vi "NC Motor GS LV.vi"() -> ()   [LabVIEW 2014]
uses:
  F:/Labview GS ver 2014/NCmotorGSLV.dll
  NCmotorGSLV.dll
  <vilib>/Instr/_visa.llb/VISA Configure Serial Port (Instr).vi
panel:
  out "SoftVer":string caption="Controller Software ver"
  in  "Baud Rate":T1(radio)=enum."9600"
  in  "StopAll":bool caption="Stop Motor"
  out "VerInfo":string caption="DLL Version"
  in  "stop":bool
  in  "VISA resource name":refnum<visa-resource-name> caption="Select Serial Port"
  in  "Serial Port":bool
  in  "M1Init":bool
  in  "M1Home":bool
  in  "M1HomeTo":T2(radio) caption="Home To"
  in  "b1SP1":bool
  in  "b1SP9":bool
  in  "b1SP8":bool
  in  "b1SP7":bool
  in  "b1SP6":bool
  in  "b1SP5":bool
  in  "b1SP4":bool
  in  "b1SP3":bool
  in  "b1SP2":bool
  in  "b1SP0":bool
  out "M1SP9":string caption="SP1"
  out "M1SP8":string caption="SP1"
  out "M1SP7":string caption="SP1"
  out "M1SP6":string caption="SP1"
  out "M1SP5":string caption="SP1"
  out "M1SP4":string caption="SP1"
  out "M1SP3":string caption="SP1"
  out "M1SP2":string caption="SP1"
  out "M1SP1":string caption="SP1"
  out "M1SP0":string caption="SP0"
  in  "StopM1":bool caption="Stop Motor"
  out "MovingM1":bool caption="Moving"
  out "ErrorM1":bool caption="Pos Error"
  out "InitM1":bool caption="Not Initialised"
  out "HomeM1":bool caption="Not Homed"
  out "ReadyM1":bool caption="Ready"
  in  "NewAccelM1":u16 caption="New Acceleration" max=5000
  in  "NewVelM1":u16 caption="New Velocity" max=5000
  out "AccelM1":string caption="Acceleration"
  out "VelM1":string caption="Velocity"
  in  "M1Send":bool
  in  "AddM1":u8=1 caption="Address" min=1 max=15 step=1 format="%x"
  out "PosM1":string caption="Position"
  in  "NewPosM1":i32 caption="New Position"
  in  "Motor1On":bool caption="Enable"
  in  "M2Init":bool
  in  "M2Home":bool
  in  "M2HomeTo":T2(radio) caption="Home To"
  out "M2SP8":string caption="SP1"
  out "M2SP9":string caption="SP1"
  out "M2SP7":string caption="SP1"
  out "M2SP6":string caption="SP1"
  out "M2SP5":string caption="SP1"
  out "M2SP4":string caption="SP1"
  out "M2SP3":string caption="SP1"
  in  "b2SP2":bool
  in  "b2SP9":bool
  in  "b2SP8":bool
  in  "b2SP7":bool
  in  "b2SP6":bool
  in  "b2SP5":bool
  in  "b2SP4":bool
  out "M2SP2":string caption="SP1"
  in  "b2SP3":bool
  in  "b2SP1":bool
  in  "b2SP0":bool
  out "M2SP1":string caption="SP1"
  out "M2SP0":string caption="SP0"
  in  "StopM2":bool caption="Stop Motor"
  in  "NewAccelM2":u16 caption="New Acceleration" max=5000
  in  "NewVelM2":u16 caption="New Velocity" max=5000
  out "AccelM2":string caption="Acceleration"
  out "VelM2":string caption="Velocity"
  in  "M2Send":bool caption="M1Send"
  out "PosM2":string caption="Position"
  in  "NewPosM2":i32 caption="New Position"
  out "MovinM2":bool caption="Moving"
  out "ErrorM2":bool caption="Pos Error"
  out "InitM2":bool caption="Not Initialised"
  out "HomeM2":bool caption="Not Home"
  out "ReadyM2":bool caption="Ready"
  in  "AddM2":u8=2 caption="Address" min=1 max=15
  in  "Motor2On":bool caption="Enable"
  in  "M3Init":bool
  in  "M3Home":bool
  in  "M3HomeTo":T2(radio) caption="Home To"
  out "M3SP9":string caption="SP1"
  out "M3SP8":string caption="SP1"
  out "M3SP7":string caption="SP1"
  out "M3SP6":string caption="SP1"
  out "M3SP5":string caption="SP1"
  out "M3SP4":string caption="SP1"
  out "M3SP3":string caption="SP1"
  in  "b3SP2":bool
  in  "b3SP9":bool
  in  "b3SP8":bool
  in  "b3SP7":bool
  in  "b3SP6":bool
  in  "b3SP5":bool
  in  "b3SP4":bool
  out "M3SP2":string caption="SP1"
  in  "b3SP3":bool
  in  "b3SP1":bool
  in  "b3SP0":bool
  out "M3SP1":string caption="SP1"
  out "M3SP0":string caption="SP0"
  in  "StopM3":bool caption="Stop Motor"
  in  "NewAccelM3":u16 caption="New Acceleration" max=5000
  in  "NewVelM3":u16 caption="New Velocity" max=5000
  out "AccelM3":string caption="Acceleration"
  out "VelM3":string caption="Velocity"
  in  "M3Send":bool caption="M1Send"
  out "PosM3":string caption="Position"
  in  "NewPosM3":i32 caption="New Position"
  out "MovinM3":bool caption="Moving"
  out "ErrorM3":bool caption="Pos Error"
  out "InitM3":bool caption="Not Initialised"
  out "HomeM3":bool caption="Not Home"
  out "ReadyM3":bool caption="Ready"
  in  "AddM3":u8=3 caption="Address" min=1 max=15
  in  "Motor3On":bool caption="Enable"
  out "error out":errorcluster
  out "RxData":string
  # "NC Motor GS LV.vi"
  # "2.  Select Baud rate"
  # "3.  Set motor address"
  # "4.  Enable motors"
  # "1.  Select COM port"
  # "5.  Open serial port"
  # "Set Points"
  # "Motor 1"
  # "Set Points"
  # "Motor 2"
  # "Set Points"
  # "Motor 3"
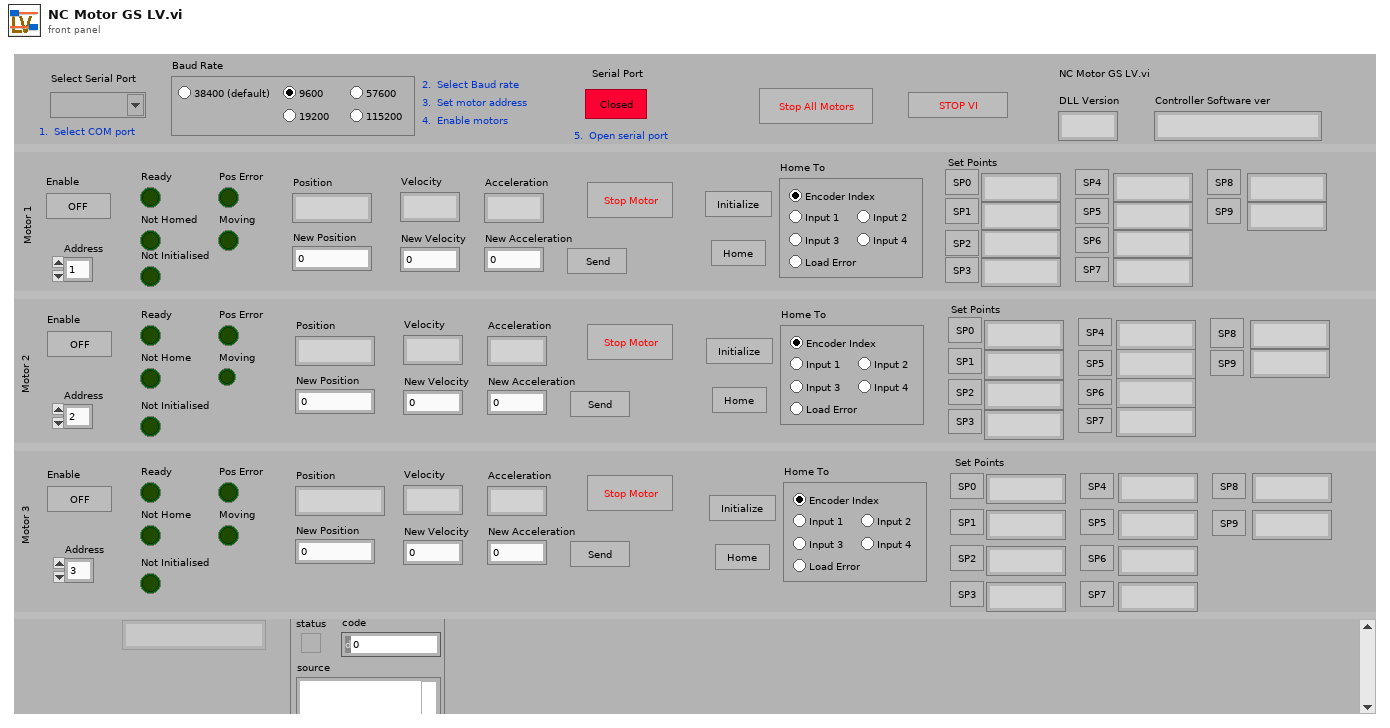
[diagram p1: front panel]
types:
  T1 = enum32{"No Selection", "9600", "19200", "38400", "57600", "115200"}
  T2 = enum32{"Enc", "Input1", "Input2", "Input3", "Input4", "Load"}
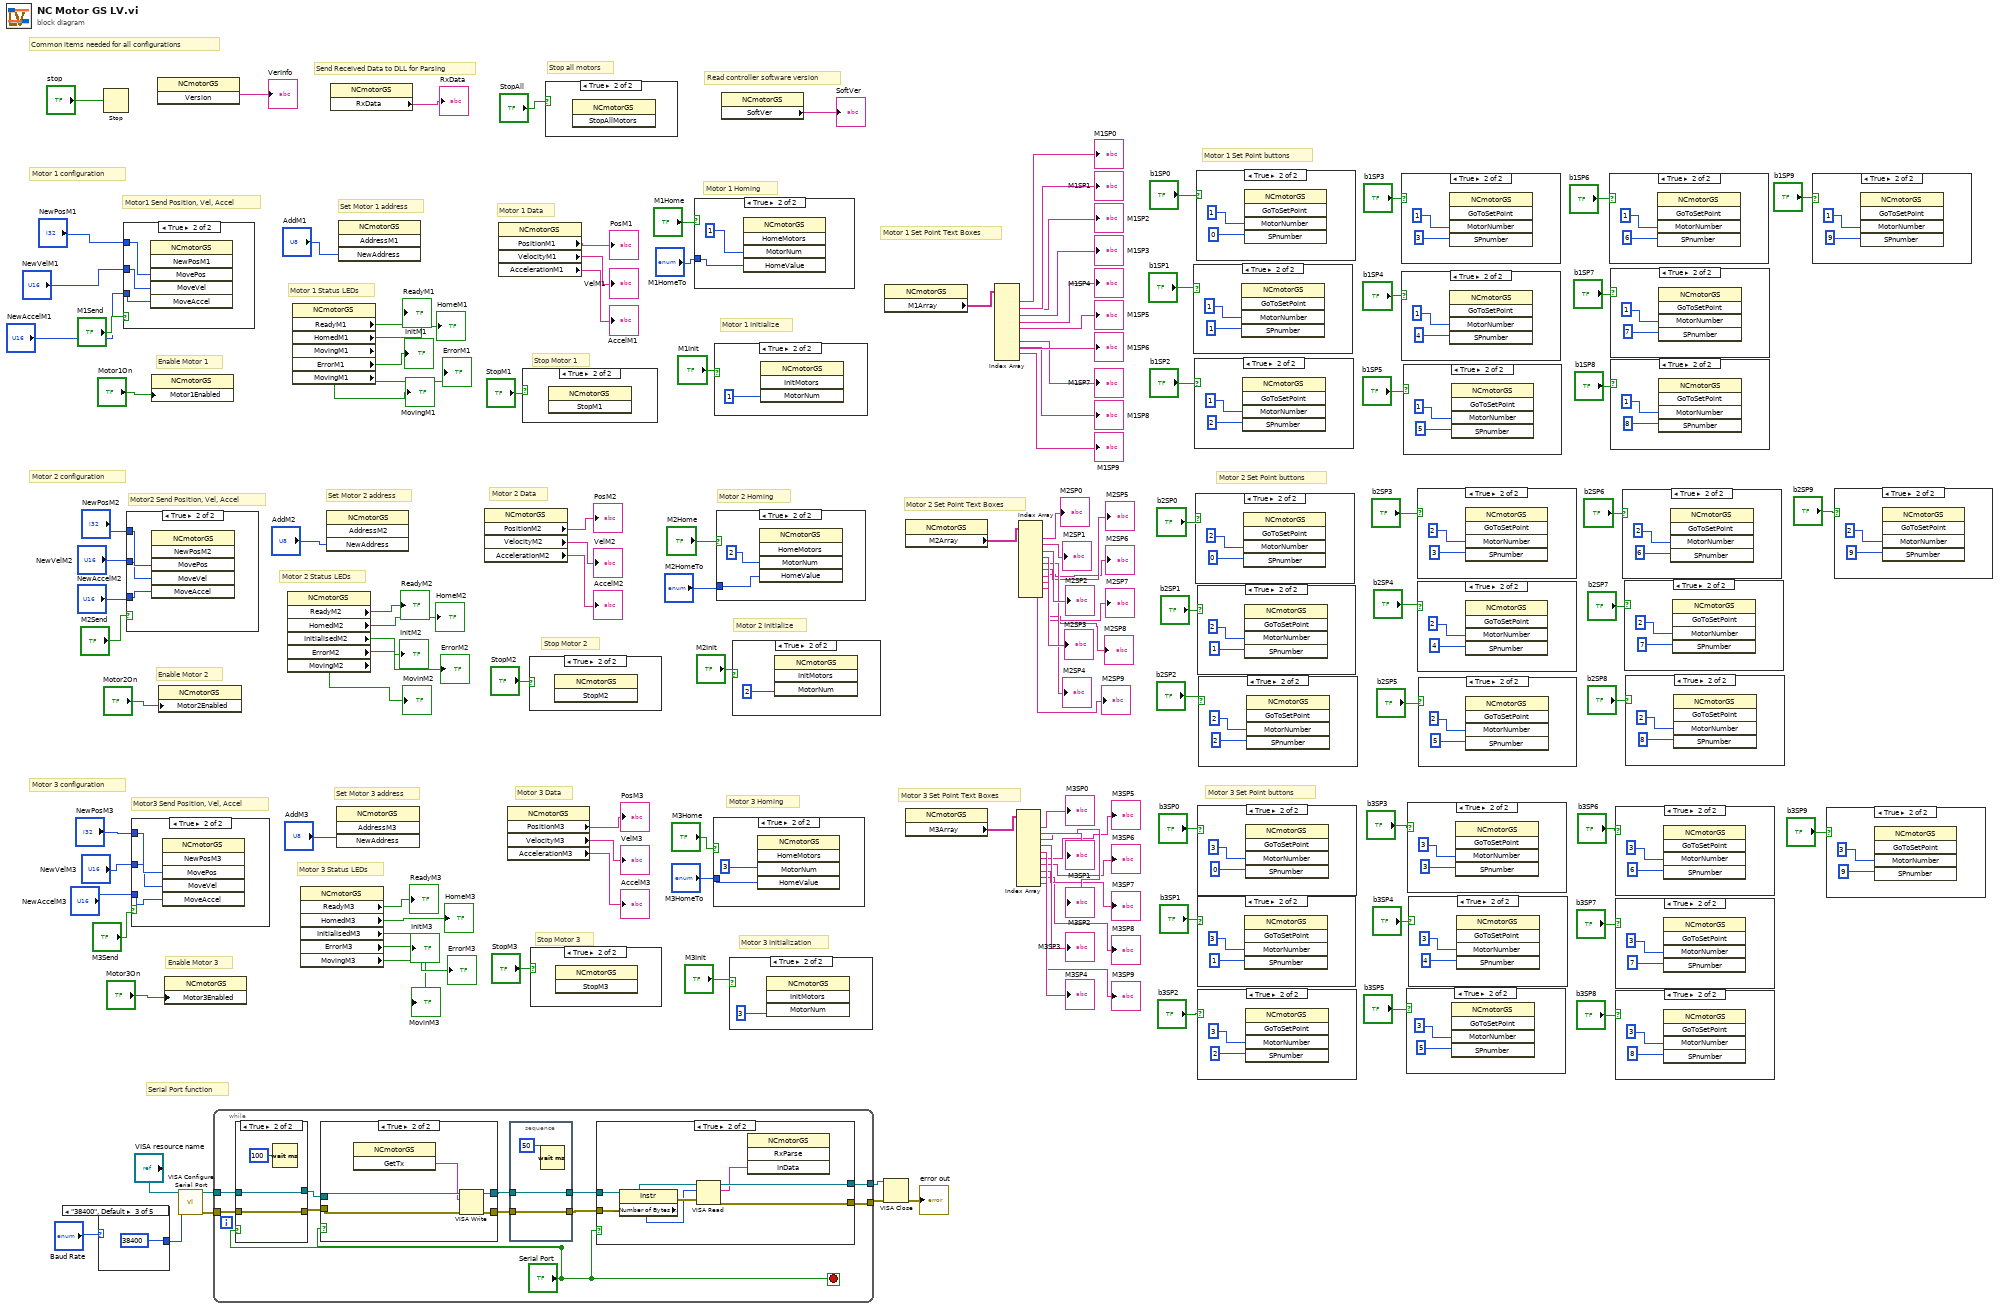
[diagram p0: block diagram]
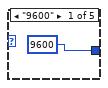
[diagram p11: hidden frame]
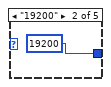
[diagram p12: hidden frame]
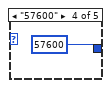
[diagram p13: hidden frame]
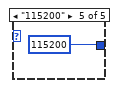
[diagram p14: hidden frame]
diagram:
  # "Read controller software version"
  # "Serial Port function"
  # "Motor 3 Homing"
  # "Motor 3 Initialization"
  # "Motor 2 Homing"
  # "Motor 2 Initialize"
  # "Motor 1 Initialize"
  # "Motor 1 Homing"
  # "Motor 3 Set Point buttons"
  # "Motor 2 Set Point buttons"
  # "Motor 1 Set Point buttons"
  # "Enable Motor 3"
  # "Enable Motor 2"
  # "Enable Motor 1"
  # "Stop Motor 1"
  # "Stop Motor 2"
  # "Stop Motor 3"
  # "Set Motor 3 address"
  # "Set Motor 2 address"
  # "Set Motor 1 address"
  # "Motor 3 configuration"
  # "Motor 1 Data"
  # "Motor 2 configuration"
  # "Motor 1 configuration"
  # "Common items needed for all configurations"
  # "Motor3 Send Position, Vel, Accel"
  # "Motor2 Send Position, Vel, Accel"
  # "Send Received Data to DLL for Parsing"
  # "Motor 2 Data"
  # "Motor 3 Data"
  # "Motor 1 Status LEDs"
  # "Motor 2 Status LEDs"
  # "Motor 3 Status LEDs"
  # "Motor 3 Set Point Text Boxes"
  # "Motor 2 Set Point Text Boxes"
  # "Motor1 Send Position, Vel, Accel"
  # "Stop all motors"
  # "Motor 1 Set Point Text Boxes"
  n1 = case shown="\"38400\", Default" "Baud Rate" {
    tunnel: [u32 9600 u32 19200 u32 38400 u32 57600 u32 115200] -> w18
    frame "9600" {
    }
    frame "19200" {
    }
    frame "38400", Default {
    }
    frame "57600" {
    }
    frame "115200" {
    }
  }
  n2 = Stop(stop? (T)="stop") -> ()
  n3 = case shown="True" "M1Send" {
    tunnel: "NewPosM1" -> [_ w138]
    tunnel: "NewVelM1" -> [_ w137]
    tunnel: "NewAccelM1" -> [_ w136]
    frame False {
    }
    frame True {
      n4 = invoke class="NCmotorGS" method="NewPosM1"("MovePos"=w138, "MoveVel"=w137, "MoveAccel"=w136) -> ()  [unwired: 3 in, 6 out]
    }
  }
  n5 = case shown="True" "M2Send" {
    tunnel: "NewPosM2" -> [_ w141]
    tunnel: "NewVelM2" -> [_ w140]
    tunnel: "NewAccelM2" -> [_ w139]
    frame False {
    }
    frame True {
      n6 = invoke class="NCmotorGS" method="NewPosM2"("MovePos"=w141, "MoveVel"=w140, "MoveAccel"=w139) -> ()  [unwired: 3 in, 6 out]
    }
  }
  n7 = case shown="True" "M3Send" {
    tunnel: "NewPosM3" -> [_ w144]
    tunnel: "NewVelM3" -> [_ w143]
    tunnel: "NewAccelM3" -> [_ w142]
    frame False {
    }
    frame True {
      n8 = invoke class="NCmotorGS" method="NewPosM3"("MovePos"=w144, "MoveVel"=w143, "MoveAccel"=w142) -> ()  [unwired: 3 in, 6 out]
    }
  }
  n9 = property class="NCmotorGS"("Motor1Enabled"="Motor1On") -> ()  [unwired: 2 in, 2 out]
  n10 = invoke class="NCmotorGS" method="Version"() -> ("Version"=→"VerInfo":string)  [unwired: 3 in, 2 out]
  n11 = property class="NCmotorGS"("Motor2Enabled"="Motor2On") -> ()  [unwired: 2 in, 2 out]
  n12 = property class="NCmotorGS"("Motor3Enabled"="Motor3On") -> ()  [unwired: 2 in, 2 out]
  n13 = call-poly "VISA Configure Serial Port"("VISA resource name"="VISA resource name", "baud rate (9600)"=w18) -> ("VISA resource name out"=w7:refnum<visa-resource-name>, "error out"=w6:errorcluster)  [unwired: 12 in]
  n14 = while {
    tunnel: w7 -> [w155]
    tunnel: w6 -> [w154]
    tunnel: [w147] -> w5
    tunnel: [w146] -> w4
    stop <- "Serial Port" stop-if-true
    n15 = case shown="True" "Serial Port" {
      tunnel: w155 -> [w177 w180]
      tunnel: w154 -> [w176 w179]
      tunnel: [w177 w180] -> w153
      tunnel: [w176 w179] -> w152
      frame False {
      }
      frame True {
        n16 = Wait (ms)(milliseconds to wait=u32 100) -> ()  [unwired: 1 out]
      }
    }
    n17 = case shown="True" "Serial Port" {
      tunnel: [w170 w175] -> w151
      tunnel: [w169 w174] -> w150
      tunnel: w153 -> [w170 w173]
      tunnel: w152 -> [w169 w172]
      frame False {
      }
      frame True {
        n18 = invoke class="NCmotorGS" method="GetTx"() -> ("GetTx"=w171:string)  [unwired: 3 in, 2 out]
        n19 = VISA Write(VISA resource name=w173, write buffer=w171, error in (no error)=w172) -> (VISA resource name out=w175:refnum<visa-resource-name>, error out=w174:errorcluster)  [unwired: 1 out]
      }
    }
    n20 = stacked-sequence {
      tunnel: w151 -> [w168]
      tunnel: w150 -> [w167]
      tunnel: [w168] -> w149
      tunnel: [w167] -> w148
      frame #0 {
        n21 = Wait (ms)(milliseconds to wait=u32 50) -> ()  [unwired: 1 out]
      }
    }
    n22 = case shown="True" "Serial Port" {
      tunnel: w149 -> [w157 w162]
      tunnel: w148 -> [w156 w161]
      tunnel: [w156 w160] -> w146
      tunnel: [w157 w159] -> w147
      frame False {
      }
      frame True {
        n23 = property on="Property Node" class="Instr"(reference=w162, error in=w161) -> (reference out=w165:refnum<visa-resource-name>, error out=w164:errorcluster, "Serial Settings:Number of Bytes at Serial Port"=w163:u32)
        n24 = VISA Read(VISA resource name=w165, byte count=w163, error in (no error)=w164) -> (VISA resource name out=w159:refnum<visa-resource-name>, read buffer=w158:string, error out=w160:errorcluster)  [unwired: 1 out]
        n25 = invoke class="NCmotorGS" method="RxParse"("InData"=w158) -> ()  [unwired: 3 in, 4 out]
      }
    }
  }
  n26 = property class="NCmotorGS"() -> ("ReadyM2"=→"ReadyM2":bool, "HomedM2"=→"HomeM2":bool, "InitialisedM2"=→"InitM2":bool, "ErrorM2"=→"ErrorM2":bool, "MovingM2"=→"MovinM2":bool)  [unwired: 2 in, 2 out]
  n27 = property class="NCmotorGS"() -> ("ReadyM1"=→"ReadyM1":bool, "HomedM1"=→"HomeM1":bool, "MovingM1"=→"InitM1":bool, "ErrorM1"=→"ErrorM1":bool, "MovingM1"=→"MovingM1":bool)  [unwired: 2 in, 2 out]
  n28 = property class="NCmotorGS"() -> ("ReadyM3"=→"ReadyM3":bool, "HomedM3"=→"HomeM3":bool, "InitialisedM3"=→"InitM3":bool, "ErrorM3"=→"ErrorM3":bool, "MovingM3"=→"MovinM3":bool)  [unwired: 2 in, 2 out]
  n29 = invoke class="NCmotorGS" method="AddressM2"("NewAddress"="AddM2") -> ()  [unwired: 3 in, 4 out]
  n30 = property class="NCmotorGS"() -> ("RxData"=→"RxData":string)  [unwired: 2 in, 2 out]
  n31 = invoke class="NCmotorGS" method="AddressM3"("NewAddress"="AddM3") -> ()  [unwired: 3 in, 4 out]
  n32 = invoke class="NCmotorGS" method="AddressM1"("NewAddress"="AddM1") -> ()  [unwired: 3 in, 4 out]
  n33 = property class="NCmotorGS"() -> ("PositionM2"=→"PosM2":string, "VelocityM2"=→"VelM2":string, "AccelerationM2"=→"AccelM2":string)  [unwired: 2 in, 2 out]
  n34 = property class="NCmotorGS"() -> ("PositionM1"=→"PosM1":string, "VelocityM1"=→"VelM1":string, "AccelerationM1"=→"AccelM1":string)  [unwired: 2 in, 2 out]
  n35 = property class="NCmotorGS"() -> ("PositionM3"=→"PosM3":string, "VelocityM3"=→"VelM3":string, "AccelerationM3"=→"AccelM3":string)  [unwired: 2 in, 2 out]
  n36 = case shown="True" "StopM1" {
    frame False {
    }
    frame True {
      n37 = invoke class="NCmotorGS" method="StopM1"() -> ()  [unwired: 3 in, 3 out]
    }
  }
  n38 = case shown="True" "StopM2" {
    frame False {
    }
    frame True {
      n39 = invoke class="NCmotorGS" method="StopM2"() -> ()  [unwired: 3 in, 3 out]
    }
  }
  n40 = case shown="True" "StopM3" {
    frame False {
    }
    frame True {
      n41 = invoke class="NCmotorGS" method="StopM3"() -> ()  [unwired: 3 in, 3 out]
    }
  }
  n42 = case shown="True" "StopAll" {
    frame False {
    }
    frame True {
      n43 = invoke class="NCmotorGS" method="StopAllMotors"() -> ()  [unwired: 3 in, 3 out]
    }
  }
  n44 = case shown="True" "M1Home" {
    tunnel: "M1HomeTo" -> [_ w181]
    frame False {
    }
    frame True {
      n45 = invoke class="NCmotorGS" method="HomeMotors"("MotorNum"=1, "HomeValue"=w181) -> ()  [unwired: 3 in, 5 out]
    }
  }
  n46 = case shown="True" "M3Home" {
    tunnel: "M3HomeTo" -> [_ w184]
    frame False {
    }
    frame True {
      n47 = invoke class="NCmotorGS" method="HomeMotors"("MotorNum"=3, "HomeValue"=w184) -> ()  [unwired: 3 in, 5 out]
    }
  }
  n48 = case shown="True" "M1Init" {
    frame False {
    }
    frame True {
      n49 = invoke class="NCmotorGS" method="InitMotors"("MotorNum"=1) -> ()  [unwired: 3 in, 4 out]
    }
  }
  n50 = case shown="True" "M2Home" {
    tunnel: "M2HomeTo" -> [_ w187]
    frame False {
    }
    frame True {
      n51 = invoke class="NCmotorGS" method="HomeMotors"("MotorNum"=2, "HomeValue"=w187) -> ()  [unwired: 3 in, 5 out]
    }
  }
  n52 = property class="NCmotorGS"() -> ("SoftVer"=→"SoftVer":string)  [unwired: 2 in, 2 out]
  n53 = case shown="True" "M3Init" {
    frame False {
    }
    frame True {
      n54 = invoke class="NCmotorGS" method="InitMotors"("MotorNum"=3) -> ()  [unwired: 3 in, 4 out]
    }
  }
  n55 = case shown="True" "M2Init" {
    frame False {
    }
    frame True {
      n56 = invoke class="NCmotorGS" method="InitMotors"("MotorNum"=2) -> ()  [unwired: 3 in, 4 out]
    }
  }
  n57 = VISA Close(VISA resource name=w5, error in (no error)=w4) -> (error out=→"error out":errorcluster)
  n58 = property class="NCmotorGS"() -> ("M1Array"=w1:string[])  [unwired: 2 in, 2 out]
  n59 = property class="NCmotorGS"() -> ("M2Array"=w62:string[])  [unwired: 2 in, 2 out]
  n60 = property class="NCmotorGS"() -> ("M3Array"=w53:string[])  [unwired: 2 in, 2 out]
  n61 = Index Array(array=w1) -> (element #1=→"M1SP0":string, element #2=→"M1SP1":string, element #3=→"M1SP2":string, element #4=→"M1SP3":string, element #5=→"M1SP4":string, element #6=→"M1SP5":string, element #7=→"M1SP6":string, element #8=→"M1SP7":string, element #9=→"M1SP8":string, element #10=→"M1SP9":string)  [unwired: 10 in]
  n62 = Index Array(array=w53) -> (element #1=→"M3SP0":string, element #2=→"M3SP1":string, element #3=→"M3SP2":string, element #4=→"M3SP3":string, element #5=→"M3SP4":string, element #6=→"M3SP5":string, element #7=→"M3SP6":string, element #8=→"M3SP7":string, element #9=→"M3SP8":string, element #10=→"M3SP9":string)  [unwired: 10 in]
  n63 = Index Array(array=w62) -> (element #1=→"M2SP0":string, element #2=→"M2SP1":string, element #3=→"M2SP2":string, element #4=→"M2SP3":string, element #5=→"M2SP4":string, element #6=→"M2SP5":string, element #7=→"M2SP6":string, element #8=→"M2SP7":string, element #9=→"M2SP8":string, element #10=→"M2SP9":string)  [unwired: 10 in]
  n64 = case shown="True" "b1SP1" {
    frame False {
    }
    frame True {
      n65 = invoke class="NCmotorGS" method="GoToSetPoint"("MotorNumber"=1, "SPnumber"=1) -> ()  [unwired: 3 in, 5 out]
    }
  }
  n66 = case shown="True" "b1SP2" {
    frame False {
    }
    frame True {
      n67 = invoke class="NCmotorGS" method="GoToSetPoint"("MotorNumber"=1, "SPnumber"=2) -> ()  [unwired: 3 in, 5 out]
    }
  }
  n68 = case shown="True" "b2SP0" {
    frame False {
    }
    frame True {
      n69 = invoke class="NCmotorGS" method="GoToSetPoint"("MotorNumber"=2, "SPnumber"=0) -> ()  [unwired: 3 in, 5 out]
    }
  }
  n70 = case shown="True" "b1SP0" {
    frame False {
    }
    frame True {
      n71 = invoke class="NCmotorGS" method="GoToSetPoint"("MotorNumber"=1, "SPnumber"=0) -> ()  [unwired: 3 in, 5 out]
    }
  }
  n72 = case shown="True" "b2SP1" {
    frame False {
    }
    frame True {
      n73 = invoke class="NCmotorGS" method="GoToSetPoint"("MotorNumber"=2, "SPnumber"=1) -> ()  [unwired: 3 in, 5 out]
    }
  }
  n74 = case shown="True" "b3SP1" {
    frame False {
    }
    frame True {
      n75 = invoke class="NCmotorGS" method="GoToSetPoint"("MotorNumber"=3, "SPnumber"=1) -> ()  [unwired: 3 in, 5 out]
    }
  }
  n76 = case shown="True" "b3SP0" {
    frame False {
    }
    frame True {
      n77 = invoke class="NCmotorGS" method="GoToSetPoint"("MotorNumber"=3, "SPnumber"=0) -> ()  [unwired: 3 in, 5 out]
    }
  }
  n78 = case shown="True" "b3SP2" {
    frame False {
    }
    frame True {
      n79 = invoke class="NCmotorGS" method="GoToSetPoint"("MotorNumber"=3, "SPnumber"=2) -> ()  [unwired: 3 in, 5 out]
    }
  }
  n80 = case shown="True" "b2SP2" {
    frame False {
    }
    frame True {
      n81 = invoke class="NCmotorGS" method="GoToSetPoint"("MotorNumber"=2, "SPnumber"=2) -> ()  [unwired: 3 in, 5 out]
    }
  }
  n82 = case shown="True" "b1SP3" {
    frame False {
    }
    frame True {
      n83 = invoke class="NCmotorGS" method="GoToSetPoint"("MotorNumber"=1, "SPnumber"=3) -> ()  [unwired: 3 in, 5 out]
    }
  }
  n84 = case shown="True" "b1SP4" {
    frame False {
    }
    frame True {
      n85 = invoke class="NCmotorGS" method="GoToSetPoint"("MotorNumber"=1, "SPnumber"=4) -> ()  [unwired: 3 in, 5 out]
    }
  }
  n86 = case shown="True" "b1SP5" {
    frame False {
    }
    frame True {
      n87 = invoke class="NCmotorGS" method="GoToSetPoint"("MotorNumber"=1, "SPnumber"=5) -> ()  [unwired: 3 in, 5 out]
    }
  }
  n88 = case shown="True" "b3SP5" {
    frame False {
    }
    frame True {
      n89 = invoke class="NCmotorGS" method="GoToSetPoint"("MotorNumber"=3, "SPnumber"=5) -> ()  [unwired: 3 in, 5 out]
    }
  }
  n90 = case shown="True" "b3SP3" {
    frame False {
    }
    frame True {
      n91 = invoke class="NCmotorGS" method="GoToSetPoint"("MotorNumber"=3, "SPnumber"=3) -> ()  [unwired: 3 in, 5 out]
    }
  }
  n92 = case shown="True" "b3SP4" {
    frame False {
    }
    frame True {
      n93 = invoke class="NCmotorGS" method="GoToSetPoint"("MotorNumber"=3, "SPnumber"=4) -> ()  [unwired: 3 in, 5 out]
    }
  }
  n94 = case shown="True" "b2SP3" {
    frame False {
    }
    frame True {
      n95 = invoke class="NCmotorGS" method="GoToSetPoint"("MotorNumber"=2, "SPnumber"=3) -> ()  [unwired: 3 in, 5 out]
    }
  }
  n96 = case shown="True" "b2SP4" {
    frame False {
    }
    frame True {
      n97 = invoke class="NCmotorGS" method="GoToSetPoint"("MotorNumber"=2, "SPnumber"=4) -> ()  [unwired: 3 in, 5 out]
    }
  }
  n98 = case shown="True" "b2SP5" {
    frame False {
    }
    frame True {
      n99 = invoke class="NCmotorGS" method="GoToSetPoint"("MotorNumber"=2, "SPnumber"=5) -> ()  [unwired: 3 in, 5 out]
    }
  }
  n100 = case shown="True" "b1SP6" {
    frame False {
    }
    frame True {
      n101 = invoke class="NCmotorGS" method="GoToSetPoint"("MotorNumber"=1, "SPnumber"=6) -> ()  [unwired: 3 in, 5 out]
    }
  }
  n102 = case shown="True" "b1SP7" {
    frame False {
    }
    frame True {
      n103 = invoke class="NCmotorGS" method="GoToSetPoint"("MotorNumber"=1, "SPnumber"=7) -> ()  [unwired: 3 in, 5 out]
    }
  }
  n104 = case shown="True" "b1SP8" {
    frame False {
    }
    frame True {
      n105 = invoke class="NCmotorGS" method="GoToSetPoint"("MotorNumber"=1, "SPnumber"=8) -> ()  [unwired: 3 in, 5 out]
    }
  }
  n106 = case shown="True" "b3SP6" {
    frame False {
    }
    frame True {
      n107 = invoke class="NCmotorGS" method="GoToSetPoint"("MotorNumber"=3, "SPnumber"=6) -> ()  [unwired: 3 in, 5 out]
    }
  }
  n108 = case shown="True" "b3SP7" {
    frame False {
    }
    frame True {
      n109 = invoke class="NCmotorGS" method="GoToSetPoint"("MotorNumber"=3, "SPnumber"=7) -> ()  [unwired: 3 in, 5 out]
    }
  }
  n110 = case shown="True" "b3SP8" {
    frame False {
    }
    frame True {
      n111 = invoke class="NCmotorGS" method="GoToSetPoint"("MotorNumber"=3, "SPnumber"=8) -> ()  [unwired: 3 in, 5 out]
    }
  }
  n112 = case shown="True" "b2SP6" {
    frame False {
    }
    frame True {
      n113 = invoke class="NCmotorGS" method="GoToSetPoint"("MotorNumber"=2, "SPnumber"=6) -> ()  [unwired: 3 in, 5 out]
    }
  }
  n114 = case shown="True" "b2SP7" {
    frame False {
    }
    frame True {
      n115 = invoke class="NCmotorGS" method="GoToSetPoint"("MotorNumber"=2, "SPnumber"=7) -> ()  [unwired: 3 in, 5 out]
    }
  }
  n116 = case shown="True" "b2SP8" {
    frame False {
    }
    frame True {
      n117 = invoke class="NCmotorGS" method="GoToSetPoint"("MotorNumber"=2, "SPnumber"=8) -> ()  [unwired: 3 in, 5 out]
    }
  }
  n118 = case shown="True" "b1SP9" {
    frame False {
    }
    frame True {
      n119 = invoke class="NCmotorGS" method="GoToSetPoint"("MotorNumber"=1, "SPnumber"=9) -> ()  [unwired: 3 in, 5 out]
    }
  }
  n120 = case shown="True" "b3SP9" {
    frame False {
    }
    frame True {
      n121 = invoke class="NCmotorGS" method="GoToSetPoint"("MotorNumber"=3, "SPnumber"=9) -> ()  [unwired: 3 in, 5 out]
    }
  }
  n122 = case shown="True" "b2SP9" {
    frame False {
    }
    frame True {
      n123 = invoke class="NCmotorGS" method="GoToSetPoint"("MotorNumber"=2, "SPnumber"=9) -> ()  [unwired: 3 in, 5 out]
    }
  }
